vi "Protocol Write.vi"(8 "error in (no error)":errorcluster, 9 "timeout":i32=10000, 10 "data":u8[](array[numeric]), 11 "protocol layer in":refnum<class "TCP Master.lvclass">) -> (0 "error out":errorcluster, 1 "timed out?":bool, 3 "protocol layer out":refnum<class "TCP Master.lvclass">)   [LabVIEW 2020, in "SubVIs.lvlib" / "TCP Master.lvclass"]
doc: "Writes to the established TCP connection stored in the class."
uses:
  <vilib>/Modbus/subvis/Protocol/TCP/TCP Master/TCP Master.lvclass
  <vilib>/Modbus/subvis/Protocol/TCP/TCP Master/TCP Master.lvclass/TCP Master.ctl
  <vilib>/Modbus/subvis/Protocol/TCP/TCP Shared Components/TCP Shared Components.lvlib
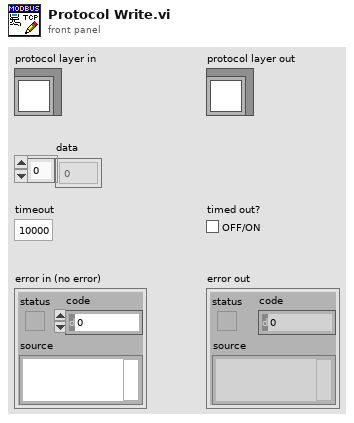
[diagram p1: front panel]
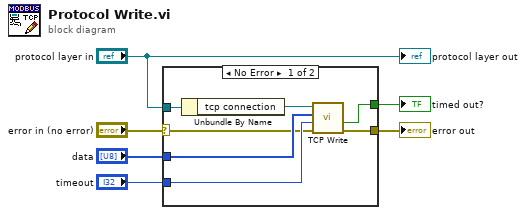
[diagram p0: block diagram]
diagram:
  n1 = case shown="No Error" "error in (no error)" {
    selector: "error in (no error)" -> [w7 w14]
    tunnel: [w13 w14] -> w6
    tunnel: [w12 _] -> w5
    tunnel: "timeout" -> [w11 _]
    tunnel: "data" -> [w10 _]
    tunnel: "protocol layer in" -> [w9 _]
    frame No Error {
      n2 = Unbundle By Name(w9) -> ("tcp connection"=w8:refnum<k5>)
      n3 = call <vilib>:"TCP Write.vi"("error in (no error)"=w7, "timeout"=w11, "data"=w10, "connection ID"=w8) -> ("error out"=w13:errorcluster, "timed out?"=w12:bool)  [unwired: 6 in]
    }
    frame Error {
    }
  }
  "error out" <- w6
  "timed out?" <- w5
  "protocol layer out" <- "protocol layer in"
